vi "rwfm_AcqRead(Wfm+OSClk).vi"(0 "Dynamic FPGA VI Reference":T1, 1 "Poll Time (ms)":u32=10, 5 "Sampling Info":T2={"Number of Channels"=4, "Sampling Rate"=5120.0, "Channels"=[], "Units"=[], "Offsets"=[]}, 9 "Samps Read per Chan":i32, 11 "error in":errorcluster, 12 "Timeout (s)":dbl=5.0) -> (3 "Time Stamp":timestamp, 4 "Dynamic FPGA VI Reference":T1, 6 "Wfm Data":waveform(sgl)[](array[waveform]), 8 "number of pulses":u32, 10 "Samples Remaining":u32, 13 "OSClkStart":dbl, 14 "OSClkStart_U32":u32, 15 "error out":errorcluster)   [LabVIEW 2017, in "cRIOWfmLib.lvlib"]
doc: "Reads waveform data from the DMA FIFO."
uses:
  <vilib>/addons/InsightCM/Devices/Shared/Cms/cRIOWfmAcq/cRIOWfmLib.lvlib
  <vilib>/addons/InsightCM/Devices/Shared/Cms/cRIOWfmAcq/subVIs/RIO Wfm Cust Ctrls/rwfm_SamplingInfo.ctl
  <vilib>/addons/InsightCM/Devices/Shared/Cms/cRIOWfmAcq/subVIs/RIO Wfm Cust Ctrls/rwfm_DynamicFPGAref2.ctl
  <vilib>/Utility/error.llb/Error Cluster From Error Code.vi
  <vilib>/rvi/errors/niLvFpgaAdjustHostInterfaceError.vi
  <vilib>/rvi/interface/nirviReadWriteControl/nirviReadWriteControl.xnode
  <vilib>/rvi/interface/nirviMethod/nirviMethod.xnode
  <vilib>/rvi/interface/Simulation/niFpgaSimulationCallBeginRW.vi
  <vilib>/FPGAPlugInAG/Dynamic/niLvFpga_ReadFifo_Dynamic.vi
  <vilib>/rvi/errors/niLvFpgaMergeErrorWithErrorCode.vi
  NiFpgaLv.dll
panel:
  out "Read Time (ms)":u32
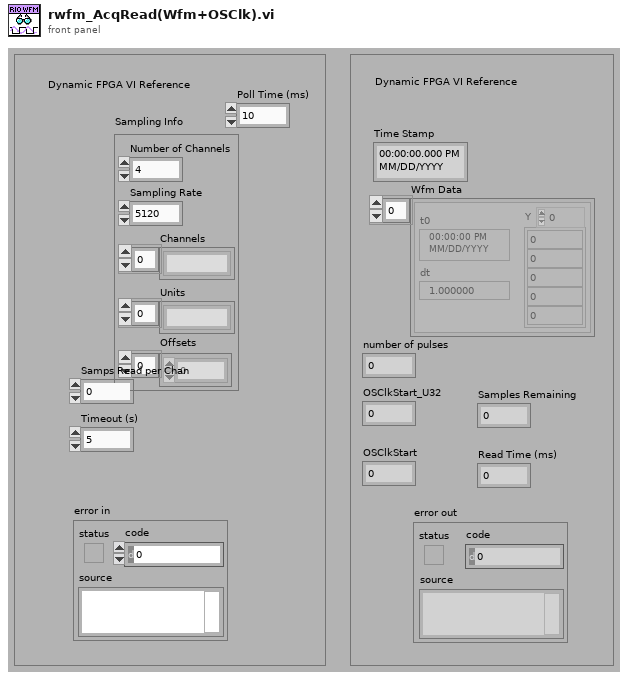
[diagram p1: front panel]
types:
  T1 = typedef "cRIOWfmLib.lvlib/rwfm_DynamicFPGAref2.ctl" = refnum<k20>
  T2 = typedef "cRIOWfmLib.lvlib/rwfm_SamplingInfo.ctl" = cluster{"Number of Channels":i32, "Sampling Rate":dbl, "Channels":string[], "Units":string[], "Offsets":sgl[]}
  T3 = typedef "rolloverState.ctl" = cluster{"prev value":u32, "total add":dbl}
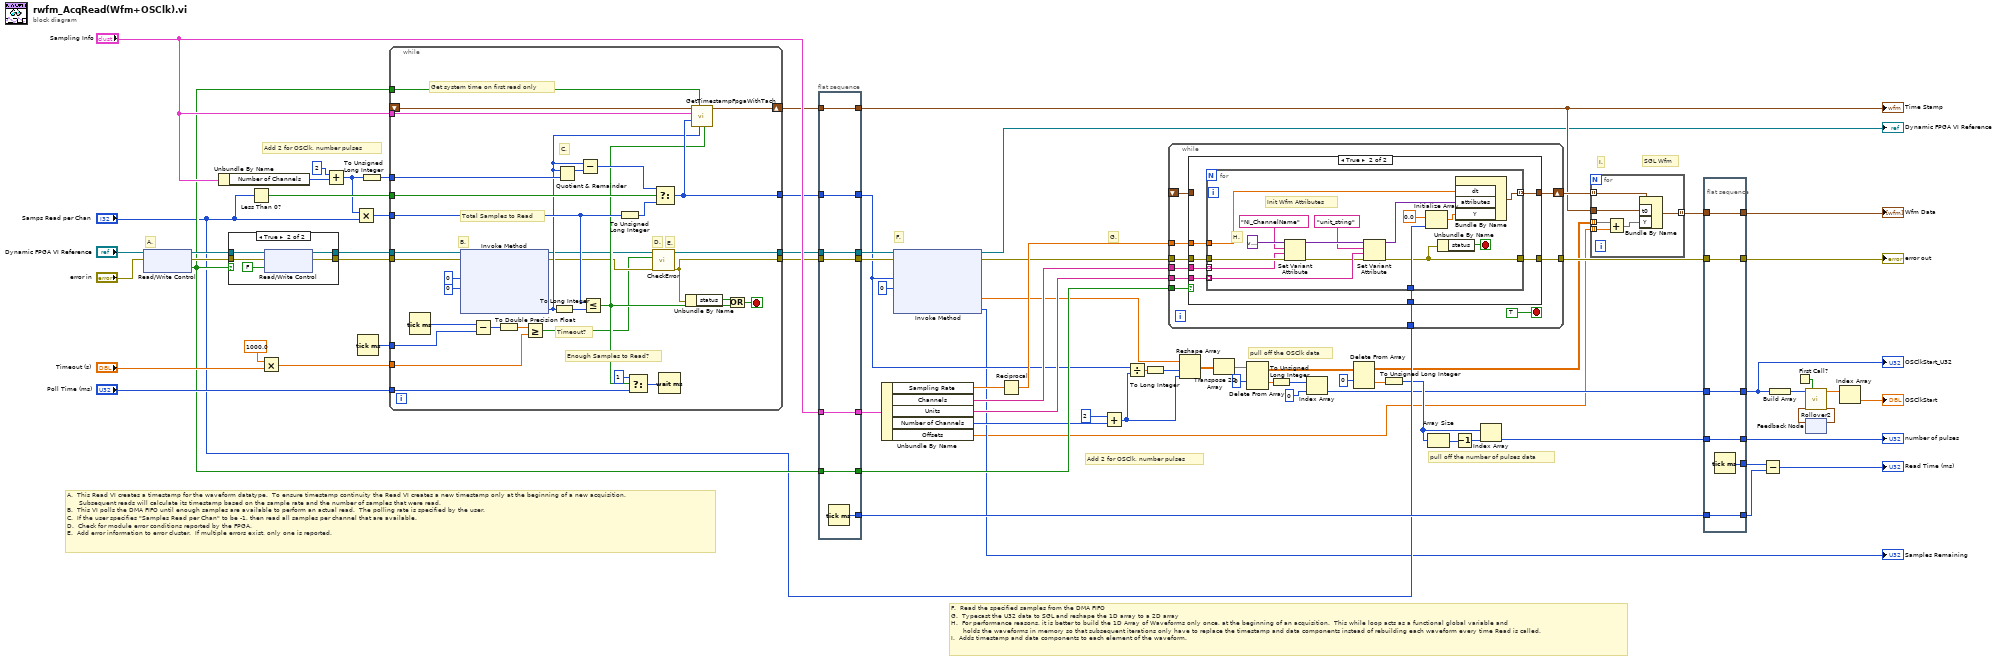
[diagram p0: block diagram]
diagram:
  # "pull off the number of pulses data"
  # "Add 2 for OSClk, number pulses"
  # "Add 2 for OSClk, number pulses"
  # "pull off the OSClk data"
  # "I."
  # "SGL Wfm"
  # "H."
  # "G."
  # "F."
  # "F.  Read the specified samples from the DMA FIFO\nG.  Typecast the U32 data to SGL and reshape the 1D array to a 2D array\nH.  For performance reasons, it is better to build the 1D Array of Waveforms only once, at the beginning of an acquisition.  This while loop acts as a functional global variable and\n      holds the waveforms in memory so that subsequent iterations only have to replace the timestamp and data components instead of rebuilding each waveform every time Read is called.\nI.  Adds timestamp and data components to each element of the waveform."
  # "A.  This Read VI creates a timestamp for the waveform datatype.  To ensure timestamp continuity the Read VI creates a new timestamp only at the beginning of a new acquisition.  \n      Subsequent reads will calculate its timestamp based on the sample rate and the number of samples that were read.\nB.  This VI polls the DMA FIFO until enough samples are available to perform an actual read.  The polling rate is specified by the user.\nC.  If the user specifies \"Samples Read per Chan\" to be -1, then read all samples per channel that are available.\nD.  Check for module error conditions reported by the FPGA.\nE.  Add error information to error cluster.  If multiple errors exist, only one is reported."
  # "A."
  n1 = xnode "Read/Write Control"("FPGA VI Reference In"="Dynamic FPGA VI Reference", "error in"="error in") -> ("FPGA VI Reference Out"=w76:T1, "error out"=w77:errorcluster, "First Read"=w39:bool)
  n2 = Unbundle By Name("Sampling Info") -> ("Number of Channels"=w24:i32)
  n3 = case shown="True" w39 {
    tunnel: w76 -> [w79 w84]
    tunnel: [w79 w83] -> w74
    tunnel: w77 -> [w78 w82]
    tunnel: [w78 w81] -> w73
    frame False {
    }
    frame True {
      n4 = xnode "Read/Write Control"("FPGA VI Reference In"=w84, "error in"=w82, "First Read"=FALSE) -> ("FPGA VI Reference Out"=w83:T1, "error out"=w81:errorcluster)
    }
  }
  n5 = Less Than 0?(x="Samps Read per Chan") -> (x < 0?=w52:bool)
  n6 = Multiply(x=1000.0 ("y"), y="Timeout (s)") -> (x*y=w69:dbl)
  n7 = Add(x=2, y=w24) -> (x+y=w23:i32)
  n8 = Multiply(x=w23, y="Samps Read per Chan") -> (x*y=w51:i32)
  n9 = Tick Count (ms)() -> (millisecond timer value=w72:u32)
  n10 = To Unsigned Long Integer(number=w23) -> (unsigned 32bit integer=w50:u32)
  n11 = while {
    tunnel: [w88] -> w57
    tunnel: [w87] -> w58
    tunnel: w39 -> [w96]
    tunnel: w74 -> [w111]
    tunnel: w73 -> [w110]
    shift-right: [w86] -> w2
    shift-left: _ -> [w85]
    tunnel: "Sampling Info" -> [w95]
    tunnel: w72 -> [w112]
    tunnel: w69 -> [w113]
    tunnel: "Poll Time (ms)" -> [w107]
    tunnel: w51 -> [w102]
    tunnel: [w94] -> w56
    tunnel: w52 -> [w105]
    tunnel: w50 -> [w101]
    stop <- w114 stop-if-true
    # "Get system time on first read only"
    # "E."
    # "C."
    # "D."
    # "B."
    # "Timeout?"
    # "Total Samples to Read"
    # "Enough Samples to Read?"
    n12 = Tick Count (ms)() -> (millisecond timer value=w109:u32)
    n13 = xnode "Invoke Method"("FPGA VI Reference In"=w111, "error in"=w110, "Number of Elements"=u32 0, "Timeout (ms)"=0) -> ("FPGA VI Reference Out"=w91:T1, "error out"=w90:errorcluster, "Elements Remaining"=w93:u32)  [unwired: 1 out]
    n14 = Subtract(x=w109, y=w112) -> (x-y=w117:u32)
    n15 = To Double Precision Float(number=w117) -> (double precision float=w116:dbl)
    n16 = Greater Or Equal?(x=w116, y=w113) -> (x >= y?=w89:bool)
    n17 = To Long Integer(number=w93) -> (32bit integer=w104:i32)
    n18 = Quotient & Remainder(x=w93, y=w101) -> (x-y*floor(x/y)=w100:u32)  [unwired: 1 out]
    n19 = Subtract(x=w93, y=w100) -> (x-y=w99:u32)
    n20 = Less Or Equal?(x=w102, y=w104) -> (x <= y?=w92:bool)
    n21 = To Unsigned Long Integer(number=w102) -> (unsigned 32bit integer=w103:u32)
    n22 = Select(t=u32 1, s=w92, f=w107) -> (s? t:f=w108:u32)
    n23 = call <vilib>:"CheckError.vi"("error in (no error)"=w90, "timeout?"=w89, "dynamic fgpa vi reference in"=w91) -> ("error out"=w88:errorcluster, "dynamic fpga vi reference out"=w87:T1)  [unwired: 7 in]
    n24 = Select(t=w99, s=w105, f=w103) -> (s? t:f=w94:u32)
    n25 = Wait (ms)(milliseconds to wait=w108) -> ()  [unwired: 1 out]
    n26 = Unbundle By Name(w88) -> ("status"=w115:bool)
    n27 = call <vilib>:"GetTimestampFpgaWithTach.vi"("Enough Samples to Read"=w92, "Elements Remaining"=w93, "First Read"=w96, "Samples to Read"=w94, "Sampling Info"=w95, "Time Stamp in"=w85) -> ("Time Stamp out"=w86:timestamp)  [unwired: 4 in, 1 out]
    n28 = Or(x=w115, y=w92) -> (x .or. y?=w114:bool)
  }
  n29 = flat-sequence {
    tunnel: [w124] -> w61
    tunnel: "Sampling Info" -> [w123]
    tunnel: [w123] -> w60
    tunnel: [w122] -> w42
    tunnel: w58 -> [w122]
    tunnel: [w121] -> w40
    tunnel: w57 -> [w121]
    tunnel: [w120] -> w36
    tunnel: w2 -> [w120]
    tunnel: [w119] -> w38
    tunnel: w56 -> [w119]
    tunnel: w39 -> [w118]
    tunnel: [w118] -> w45
    frame #0 {
      n30 = Tick Count (ms)() -> (millisecond timer value=w124:u32)
    }
  }
  n31 = Unbundle By Name(w60) -> ("Sampling Rate"=w67:dbl, "Channels"=w53:string[], "Units"=w54:string[], "Number of Channels"=w9:i32, "Offsets"=w1:sgl[])
  n32 = xnode "Invoke Method"("FPGA VI Reference In"=w42, "error in"=w40, "Number of Elements"=w38, "Timeout (ms)"=0) -> ("FPGA VI Reference Out"=→"Dynamic FPGA VI Reference":T1, "error out"=w41:errorcluster, "Data"=w34:sgl[], "Elements Remaining"=→"Samples Remaining":u32)
  n33 = Reciprocal(x=w67) -> (1/x=w66:dbl)
  n34 = Add(x=2, y=w9) -> (x+y=w21:i32)
  n35 = Divide(x=w38, y=w21) -> (x/y=w49:dbl)
  n36 = To Long Integer(number=w49) -> (32bit integer=w48:i32)
  n37 = while {
    tunnel: w66 -> [w134]
    tunnel: w41 -> [w133]
    tunnel: [w132] -> w55
    tunnel: w54 -> [w131]
    tunnel: w53 -> [w130]
    shift-right: [w129] -> w47
    shift-left: _ -> [w127]
    tunnel: w45 -> [w126]
    tunnel: "Samps Read per Chan" -> [w125]
    stop <- TRUE stop-if-true
    n38 = case shown="True" w126 {
      tunnel: w134 -> [_ w143]
      tunnel: w133 -> [w136 w142]
      tunnel: [w136 w141] -> w132
      tunnel: w131 -> [_ w140]
      tunnel: w130 -> [_ w139]
      tunnel: [w135 w138] -> w129
      tunnel: w127 -> [w135 _]
      tunnel: w125 -> [_ w137]
      frame False {
      }
      frame True {
        n39 = for {
          tunnel: w143 -> [w159]
          tunnel: [w158] -> w138 mode=indexing
          tunnel: w140 -> [w157] mode=indexing
          tunnel: w142 -> [w156]
          tunnel: [w144] -> w141
          tunnel: w139 -> [w149] mode=indexing
          tunnel: w137 -> [w146]
          stop <- w155 stop-if-true
          # "Init Wfm Attributes"
          n40 = Set Variant Attribute(Variant=variant ("variant out"), name="NI_ChannelName", value=w149, error in=w156) -> (Variant out=w153:variant, error out=w154:errorcluster)  [unwired: 1 out]
          n41 = Set Variant Attribute(Variant=w153, name="unit_string", value=w157, error in=w154) -> (Variant out=w145:variant, error out=w144:errorcluster)  [unwired: 1 out]
          n42 = Initialize Array(sgl 0.0, w146) -> (w147:sgl[])
          n43 = Unbundle By Name(w144) -> ("status"=w155:bool)
          n44 = Bundle By Name("dt"=w159, "attributes"=w145, "Y"=w147) -> (w158:waveform(sgl))  [unwired: 1 out]
        }
      }
    }
  }
  n45 = Reshape Array(w34, w48, w21) -> (w44:sgl[][])
  n46 = Transpose 2D Array(2D array=w44) -> (transposed array=w33:sgl[][])
  n47 = Delete From Array(array=w33, index (row)=0) -> (deleted portion=w30:sgl[], array with subset deleted=w18:sgl[][])  [unwired: 2 in]
  n48 = To Unsigned Long Integer(number=w30) -> (unsigned 32bit integer=w29:u32[])
  n49 = Index Array(array=w29, index=0) -> (element=w7:u32)
  n50 = Delete From Array(array=w18, index (row)=0) -> (deleted portion=w16:sgl[], array with subset deleted=w17:sgl[][])  [unwired: 2 in]
  n51 = To Unsigned Long Integer(number=w16) -> (unsigned 32bit integer=w15:u32[])
  n52 = Array Size(array=w15) -> (size(s)=w13:i32)
  n53 = Decrement(x=w13) -> (x-1=w14:i32)
  n54 = Index Array(array=w15, index=w14) -> (element=w5:u32)
  n55 = for {
    tunnel: w47 -> [w165] mode=indexing
    tunnel: w36 -> [w164]
    tunnel: [w163] -> w46 mode=indexing
    tunnel: w17 -> [w162] mode=indexing
    tunnel: w1 -> [w160] mode=indexing
    n56 = Add(x=w162, y=w160) -> (x+y=w161:sgl[])
    n57 = Bundle By Name(cluster=w165, "t0"=w164, "Y"=w161) -> (w163:waveform(sgl))
  }
  n58 = flat-sequence {
    tunnel: w55 -> [w168]
    tunnel: [w171] -> w62
    tunnel: w46 -> [w171]
    tunnel: [w170] -> w65
    tunnel: w61 -> [w169]
    tunnel: [w169] -> w64
    tunnel: [w168] -> w8
    tunnel: [w167] -> w6
    tunnel: w7 -> [w167]
    tunnel: [w166] -> w4
    tunnel: w5 -> [w166]
    frame #0 {
      n59 = Tick Count (ms)() -> (millisecond timer value=w170:u32)
    }
  }
  n60 = Subtract(x=w65, y=w64) -> (x-y=→"Read Time (ms)":u32)
  n61 = Build Array(w6) -> (w28:u32[])
  n62 = First Call?() -> (First Call?: T/F=w25:bool)
  n63 = feedback #1() -> (w11:T3)  [unwired: 1 in]
  n64 = call <vilib>:"Rollover2.vi"("reset"=w25, "rollover state"=w11, "counter"=w28) -> ("rollover state"=w12:T3, "counter"=w27:dbl[])  [unwired: 7 in]
  n65 = feedback-in #1(w12) -> ()
  n66 = Index Array(array=w27) -> (element=→"OSClkStart":dbl)  [unwired: 1 in]
  "error out" <- w8
  "Wfm Data" <- w62
  "Time Stamp" <- w36
  "OSClkStart_U32" <- w6
  "number of pulses" <- w4
